vi "Digital OUT Valves.vi"() -> ()   [LabVIEW 2014]
uses:
  <vilib>/DAQmx/create/channels.llb/DAQmx Create Channel (DO-Digital Output).vi
  <vilib>/DAQmx/read.llb/DAQmx Read (Digital 1D Bool NChan 1Samp 1Line).vi
  <vilib>/DAQmx/write.llb/DAQmx Write (Digital 1D Bool NChan 1Samp 1Line).vi
panel:
  in  "Valve 2":bool
  out "error out":errorcluster
  in  "Valve 1":bool
  in  "stop":bool
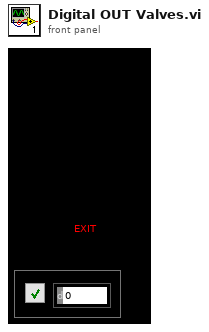
[diagram p1: front panel]
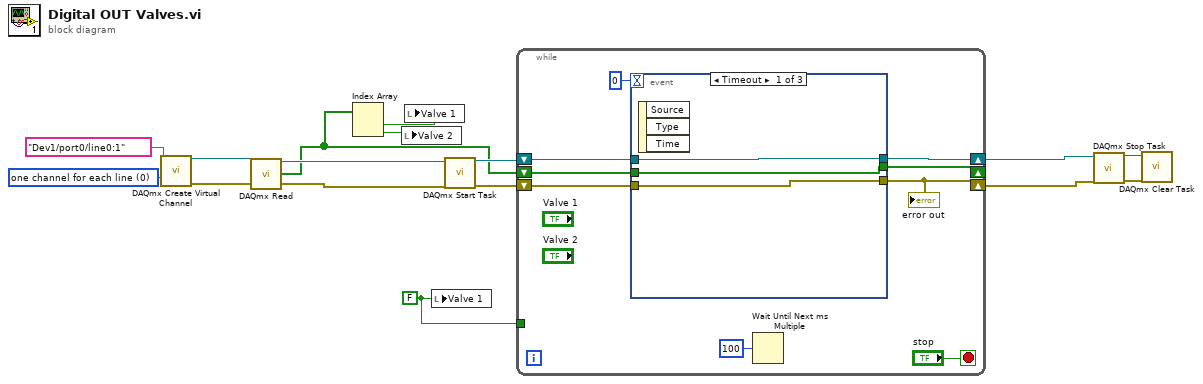
[diagram p0: block diagram]
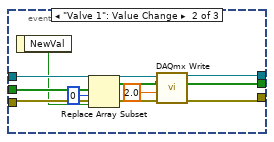
[diagram p2: hidden frame]
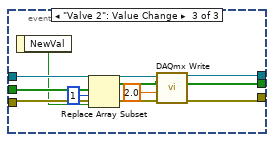
[diagram p3: hidden frame]
diagram:
  w9 = 0 items=["one channel for each line", "one channel for all lines"] ("line grouping")
  w13 = FALSE ("Turn ON")
  n1 = call-poly <vilib>:"DAQmx Create Virtual Channel.vi"("lines"=tag "Dev1/port0/line0:1", "line grouping"=w9) -> ("task out"=w11:refnum<k21>, "error out"=w10:errorcluster)  [unwired: 12 in]
  n2 = call-poly <vilib>:"DAQmx Read.vi"("task/channels in"=w11) -> ("task out"=w6:refnum<k21>, "data"=w3:bool[])  [unwired: 12 in, 1 out]
  n3 = Index Array(array=w3) -> (element #1=w1:bool, element #2=w2:bool)  [unwired: 2 in]
  n4 = local write "Valve 2"(w2) -> ()
  n5 = local write "Valve 1"(w1) -> ()
  n6 = local write "Valve 1"(w13) -> ()
  n7 = call <vilib>:"DAQmx Start Task.vi"("task/channels in"=w6, "error in"=w10) -> ("task out"=w5:refnum<k21>, "error out"=w4:errorcluster)  [unwired: 12 in]
  n8 = while {
    shift-right: [w21] -> w8
    shift-left: w5 -> [w22]
    shift-right: [w19] -> w7
    shift-left: w4 -> [w20]
    tunnel: w13 -> [_]
    shift-right: [w16] -> _
    shift-left: w3 -> [w17]
    stop <- "stop" stop-if-true
    n9 = event shown="[0] Timeout" {
      selector: _ -> [_ _ _]
      dyn-events: _ -> [_ _ _]
      timeout: 0 -> [_ _ _]
      tunnel: w22 -> [w27 w36 w45]
      tunnel: [w27 w35 w44] -> w21
      tunnel: w20 -> [w26 w33 w42]
      tunnel: [w26 w34 w43] -> w19
      tunnel: w17 -> [w25 w31 w40]
      tunnel: [w25 w28 w37] -> w16
      event Timeout {
        n10 = event-data() -> ()  [unwired: 1 in, 3 out]
      }
      event "Valve 1": Value Change {
        n11 = event-data() -> ("NewVal"=w29:bool)  [unwired: 1 in]
        n12 = Replace Array Subset(array=w31, new element=w29, index=0) -> (w28:bool[])
        n13 = call-poly <vilib>:"DAQmx Write.vi"("task/channels in"=w36, "data"=w28, "timeout"=2.0, "error in"=w33) -> ("task out"=w35:refnum<k21>, "error out"=w34:errorcluster)  [unwired: 9 in, 1 out]
      }
      event "Valve 2": Value Change {
        n14 = event-data() -> ("NewVal"=w38:bool)  [unwired: 1 in]
        n15 = Replace Array Subset(array=w40, new element=w38, index=1) -> (w37:bool[])
        n16 = call-poly <vilib>:"DAQmx Write.vi"("task/channels in"=w45, "data"=w37, "timeout"=2.0, "error in"=w42) -> ("task out"=w44:refnum<k21>, "error out"=w43:errorcluster)  [unwired: 9 in, 1 out]
      }
    }
    "error out" <- w19
    n17 = Wait Until Next ms Multiple(millisecond multiple=u32 100) -> ()  [unwired: 1 out]
  }
  n18 = call <vilib>:"DAQmx Stop Task.vi"("task/channels in"=w8, "error in"=w7) -> ("task out"=w15:refnum<k21>, "error out"=w14:errorcluster)  [unwired: 12 in]
  n19 = call <vilib>:"DAQmx Clear Task.vi"("task in"=w15, "error in"=w14) -> ()  [unwired: 13 in, 1 out]
